vi "GCMPlugin_GetPluginName.vi"(8 "error in (no error)":errorcluster, 11 "_BasicVIDocumentation in":refnum<class "GCMIconEditor.lvclass">) -> (0 "error out":errorcluster, 2 "PluginName":string, 3 "_BasicVIDocumentation out":refnum<class "GCMIconEditor.lvclass">)   [LabVIEW 2014, in "GCMIconEditor.lvlib" / "GCMIconEditor.lvclass"]
uses:
  GCMIconEditor.lvclass
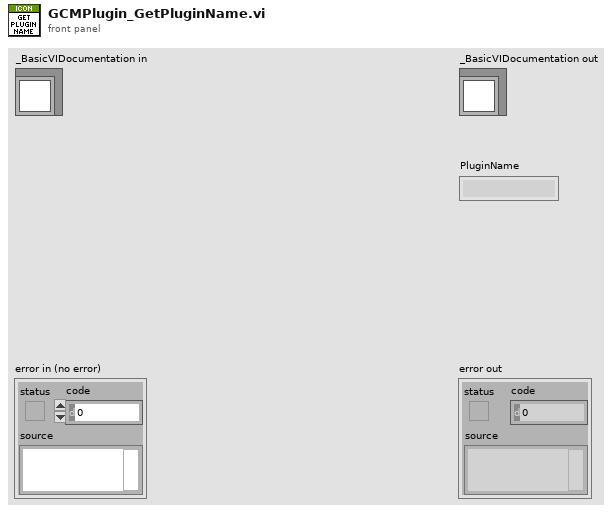
[diagram p1: front panel]
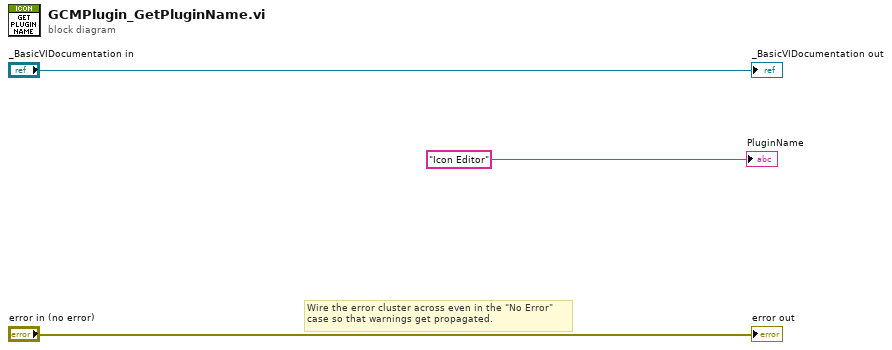
[diagram p0: block diagram]
diagram:
  # "Wire the error cluster across even in the \"No Error\"\ncase so that warnings get propagated."
  "error out" <- "error in (no error)"
  "_BasicVIDocumentation out" <- "_BasicVIDocumentation in"
  "PluginName" <- "Icon Editor"
